vi "Z6_Beamline_Chief.destructor.vi"(0 "i ref in":refnum<vi>, 5 "error in(no error)":errorcluster) -> (19 "error out":errorcluster)   [LabVIEW 2014, in "Z6_Beamline_Chief.lvlib"]
doc: "This is the destructor of a class.\n\nLicense Agreement for this software:\n\nCopyright (C)\nGesellschaft für Schwerionenforschung, GSI\nPlanckstr. 1\n64291 Darmstadt\nGermany\n\nContact: D.Beck@gsi.de \n\nThis program is free software; you can redistribute it and/or modify it under the terms of the \nGNU General Public License as published by the Free Software Foundation; either version 2 of \nthe license, or (at your option) any later version.\n\nThis program is distributed in the hope that it will be useful, but WITHOUT ANY WARRANTY; \nwithout even the implied warranty of MERCHANTABILITY or FITNESS FOR A PARTICULAR PURPOSE. See the GNU General License for more details (http://www.gnu.org).\n\nGesellschaft für Schwerionenforschung, GSI\nPlanckstr. 1, 64291 Darmstadt, Germany\nFor all questions and ideas contact: M.Richter@gsi.de, H.Brand@gsi.de or D.Beck@gsi.de.\nLast update: 16-JUN-2004"
uses:
  Z6_Beamline_Chief.lvlib
  CSlibraries-extern/DimLVEvent/LVDimInterface/LVDimInterface.lvlib
  Z6_Beamline/Z6_Beamline.lvlib
  PH_BL-Master/PH_BL-Master.lvlib
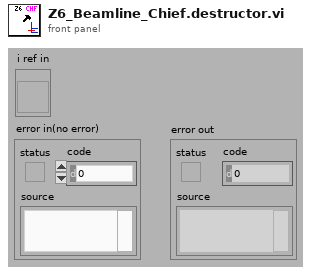
[diagram p1: front panel]
types:
  T1 = typedef "Z6_Beamline_Chief.lvlib/Z6_Beamline_Chief.i attribute.ctl" = cluster{"R2S Service ID":i32}
  T2 = enum16{"SetAttribute", "GetAttribute", "CreateAttribute", "DestroyAttribute", "DestroyAllAtributes"}
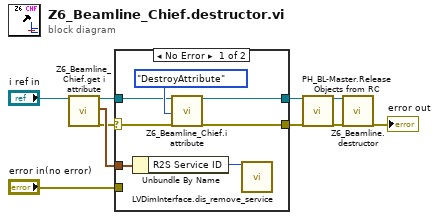
[diagram p0: block diagram]
diagram:
  n1 = call "Z6_Beamline_Chief.get i attribute.vi"("i ref in"="i ref in") -> ("i ref out"=w8:refnum<vi>, "i attribute"=w10:T1, "error out"=w7:errorcluster)  [unwired: 16 in]
  n2 = case shown="No Error" w7 {
    selector: w7 -> [w12 _]
    tunnel: w10 -> [w16 _]
    tunnel: w8 -> [w13 w19]
    tunnel: [w15 w19] -> w3
    tunnel: [w14 w18] -> w1
    tunnel: "error in(no error)" -> [_ w18]
    frame No Error {
      n3 = Unbundle By Name(w16) -> ("R2S Service ID"=w11:i32)
      n4 = call "Z6_Beamline_Chief.i attribute.vi"("VI Refnum"=w13, "Action"=T2."DestroyAttribute", "error in (no error)"=w12) -> ("VI Refnum out"=w15:refnum<vi>, "error out"=w14:errorcluster)  [unwired: 14 in, 1 out]
      n5 = call "LVDimInterface.dis_remove_service.vi"("my_serviceID"=w11) -> ()  [unwired: 18 in, 1 out]
    }
    frame Error {
    }
  }
  n6 = call "PH_BL-Master.Release Objects from RC.vi"("VI in"=w3, "error in (no error)"=w1) -> ("VI out"=w4:refnum<vi>, "error out"=w2:errorcluster)  [unwired: 16 in]
  n7 = call "Z6_Beamline.destructor.vi"("i ref in"=w4, "error in(no error)"=w2) -> ("error out"=→"error out":errorcluster)  [unwired: 17 in]
